vi "登录验证.vi"(1 "密   码":string, 2 "用户名":string) -> (0 "是否登录":bool)   [LabVIEW 2023]
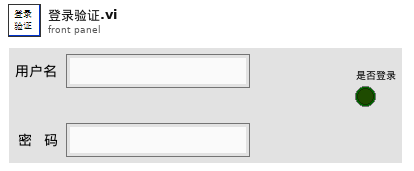
[diagram p1: front panel]
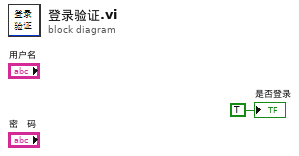
[diagram p0: block diagram]
diagram:
  "是否登录" <- TRUE ("是否登录")
